vi "Write SA Pin.vi"(8 "error in (no error)":errorcluster, 10 "SA Pin":string, 11 "SpecAn_CHP in":refnum<class "SpecAn_CHP.lvclass">) -> (0 "error out":errorcluster, 3 "SpecAn_CHP out":refnum<class "SpecAn_CHP.lvclass">)   [LabVIEW 2018, in "SeqAuto Evaluations.lvlib" / "SpecAn_CHP.lvclass"]
uses:
  SpecAn_CHP.lvclass
  SpecAn_CHP.lvclass/SpecAn_CHP.ctl
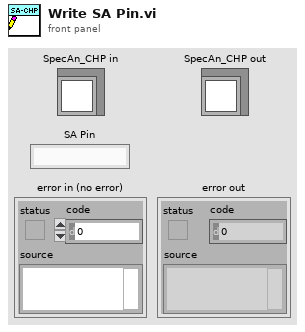
[diagram p1: front panel]
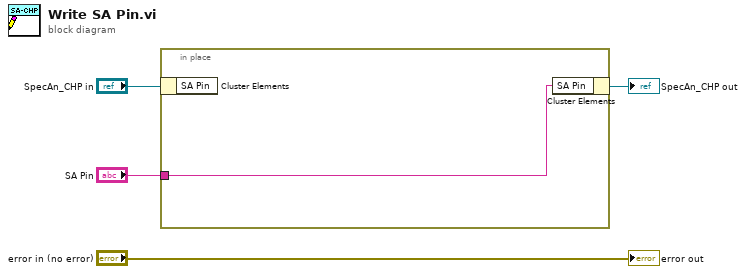
[diagram p0: block diagram]
diagram:
  n1 = in-place {
    in-place-border: "SA Pin" -> [w5]
    n2 = in-place-cluster #1("SpecAn_CHP in") -> ()  [unwired: 1 out]
    n3 = in-place-cluster #1("SA Pin"=w5) -> (→"SpecAn_CHP out":refnum<class "SpecAn_CHP.lvclass">)
  }
  "error out" <- "error in (no error)"
